vi "Test Get TSInstall by Version.vi"() -> ()   [LabVIEW 2025]
doc: "Tests fetching a specific installation."
uses:
  src/TSDiscovery Mock/TSDiscovery Mock.lvclass
  src/Type Definitions/Architecture--enum.ctl
  <vilib>/addons/_JKI Toolkits/Caraya/classes/Assert/Assert True.vi
  <vilib>/addons/_JKI Toolkits/Caraya/classes/Test/Test.lvclass
  <vilib>/addons/_JKI Toolkits/Caraya/classes/Assert/Assert.lvclass
panel:
  out "error out":errorcluster
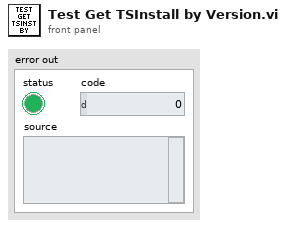
[diagram p1: front panel]
types:
  T1 = typedef "Architecture--enum.ctl" = enum16{"32bit", "64bit"}
  T2 = typedef "TSInstall--cluster.ctl" = cluster{"Version":string, "Architecture":T1, "Version Key":string, "ID":string}
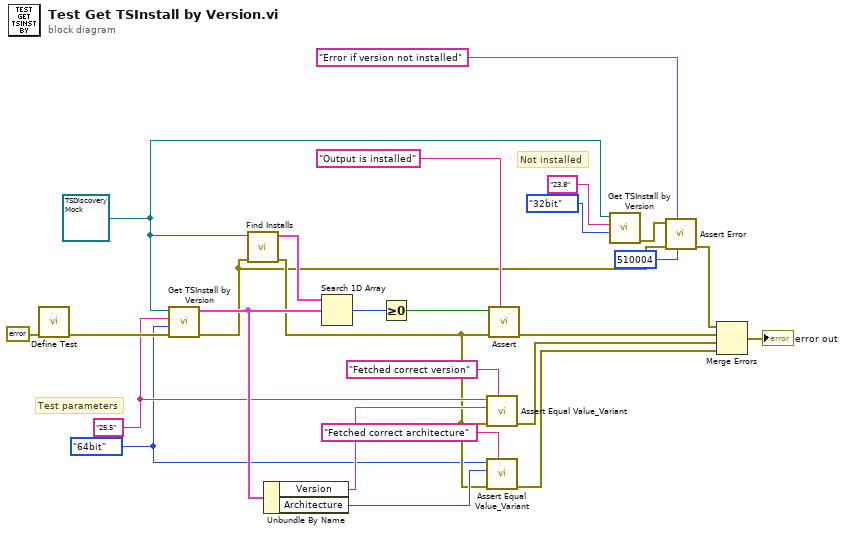
[diagram p0: block diagram]
diagram:
  w1 = Architecture--enum."64bit" ("Architecture")
  w18 = "25.5" ("Version")
  w10 = refnum<class "TSDiscovery Mock.lvclass"> refnum ("TSDiscovery Mock.lvclass")
  # "Not installed"
  # "Test parameters"
  n1 = call <vilib>:"Define Test.vi"("error in (no error)"=errorcluster {"status"=FALSE, "code"=0, "source"=""}) -> ("error out"=w23:errorcluster)  [unwired: 9 in, 1 out]
  n2 = call "Get TSInstall by Version.vi"("error in"=w23, "Architecture"=w1, "Version"=w18, "ITSDiscovery in"=w10) -> ("error out"=w3:errorcluster, "TSInstall Out"=w19:T2)  [unwired: 6 in]
  n3 = call-dynamic "Find Installs.vi"("error in"=w3, "TSDiscovery Mock in"=w10) -> ("error out"=w15:errorcluster, "TSInstalls Out"=w22:T2[])  [unwired: 8 in]
  n4 = Unbundle By Name(w19) -> ("Version"=w17:string, "Architecture"=w16:T1)
  n5 = Search 1D Array(1D array=w22, element=w19) -> (index of element=w21:i32)  [unwired: 1 in]
  n6 = Greater Or Equal To 0?(x=w21) -> (x >= 0?=w20:bool)
  n7 = call <vilib>:"Assert Equal Value_Variant.vi"("Label"="Fetched correct version", "error in (no error)"=w15, "Actual"=w17, "Expected"=w18) -> ("error out"=w13:errorcluster)  [unwired: 6 in, 1 out]
  n8 = call <vilib>:"Assert Equal Value_Variant.vi"("Label"="Fetched correct architecture", "error in (no error)"=w15, "Actual"=w16, "Expected"=w1) -> ("error out"=w14:errorcluster)  [unwired: 6 in, 1 out]
  n9 = call-poly <vilib>:"Assert.vi"("Label"="Output is installed" ("Label (VI Title)"), "error in (no error)"=w15, "True?"=w20) -> ("error out"=w25:errorcluster)  [unwired: 7 in, 1 out]
  n10 = call "Get TSInstall by Version.vi"("Architecture"=Architecture--enum."32bit", "Version"="23.8", "ITSDiscovery in"=w10) -> ("error out"=w7:errorcluster)  [unwired: 7 in, 1 out]
  n11 = call <vilib>:"Assert Error.vi"("error code (1)"=510004, "Label"="Error if version not installed", "error in (no error)"=w3, "Error?"=w7) -> ("error out"=w5:errorcluster)  [unwired: 6 in, 1 out]
  n12 = Merge Errors(w5, w25, w13, w14) -> (→"error out":errorcluster)
